vi "Write Register.vi"   [LabVIEW 2020, in "SLSC.lvlib"]
doc: "Writes <B>data</B> to the <B>register address</B> of the specified <B>device</B>."
uses:
  <vilib>/SLSC/SLSC.lvlib
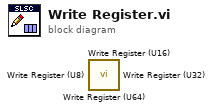
[diagram p0: block diagram]
diagram:
  n1 = call <vilib>:"Write Register (U64).vi"() -> ()  [unwired: 12 in, 4 out]
  n2 = call <vilib>:"Write Register (U16).vi"() -> ()  [unwired: 12 in, 4 out]
  n3 = call <vilib>:"Write Register (U8).vi"() -> ()  [unwired: 12 in, 4 out]
  n4 = call <vilib>:"Write Register (U32).vi"() -> ()  [unwired: 12 in, 4 out]
